vi "Display Error.vi"(8 "error in (no error)":errorcluster, 9 "LabActor Error":T1, 10 "Error message":string, 11 "LabActor in":refnum<class "LabActor.lvclass">) -> (0 "error out":errorcluster, 3 "LabActor out":refnum<class "LabActor.lvclass">)   [LabVIEW 2020, in "LabActor.lvclass"]
uses:
  LabActor.lvclass
  Template Module/LabActor Error.ctl
  LabActor.lvclass/LabActor.ctl
  Controllers/Application Controller/Application Controller.lvclass
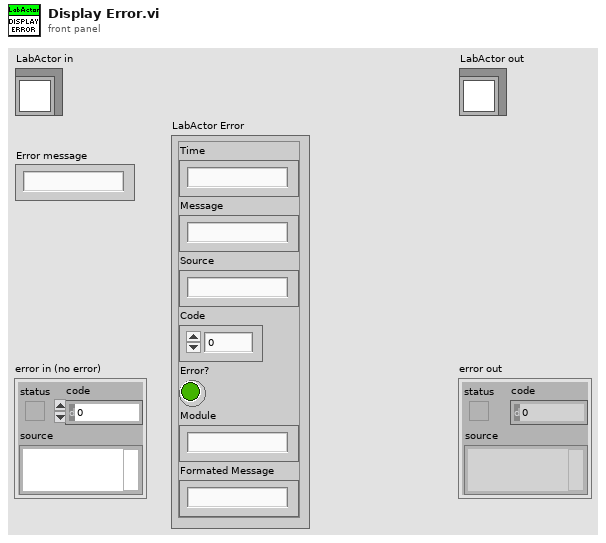
[diagram p1: front panel]
types:
  T1 = typedef "LabActor Error.ctl" = cluster{"Time":string, "Message":string, "Source":string, "Code":i32, "Error?":bool, "Module":string, "Formated Message":string}
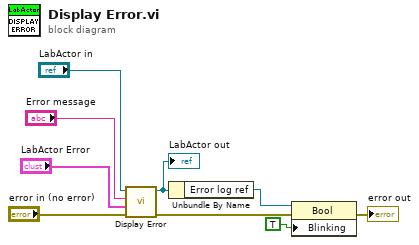
[diagram p0: block diagram]
diagram:
  n1 = call-parent "Display Error.vi"("error in (no error)"="error in (no error)", "LabActor Error"="LabActor Error", "Error message"="Error message", "Application Controller in"="LabActor in") -> ("error out"=w2:errorcluster, "Application Controller out"=w5:refnum<class "LabActor.lvclass">)  [unwired: 6 in]
  "LabActor out" <- w5
  n2 = Unbundle By Name(w5) -> ("Error log ref"=w4:refnum<vi>)
  n3 = property class="Bool"(reference=w4, error in=w2, "Blinking"=TRUE) -> (error out=→"error out":errorcluster)  [unwired: 1 out]
